vi "5.5.vi"() -> ()   [LabVIEW 2017]
panel:
  out "波形图表":dynamicdata(graph)
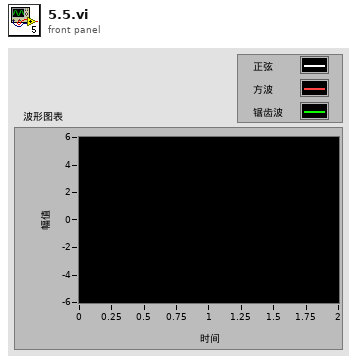
[diagram p1: front panel]
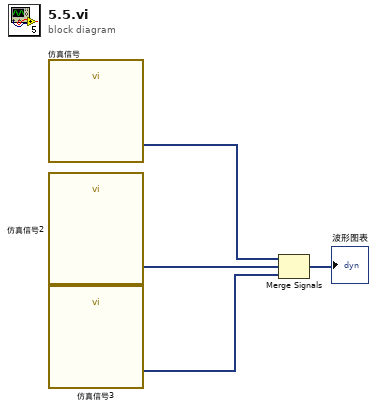
[diagram p0: block diagram]
diagram:
  n1 = call "仿真信号"() -> ("正弦"=w3:dynamicdata)  [unwired: 14 in, 1 out]
  n2 = call "仿真信号2"() -> ("方波"=w2:dynamicdata)  [unwired: 14 in, 1 out]
  n3 = call "仿真信号3"() -> ("锯齿波"=w4:dynamicdata)  [unwired: 14 in, 1 out]
  n4 = Merge Signals(w3, w2, w4) -> (→"波形图表":dynamicdata)
